vi "UserEventDemo.vi"() -> ()   [LabVIEW 2014]
panel:
  out "progress":i32(slide) scale=0.0..100.0
  out "Msg":string
  in  "ButtonB":bool
  in  "ButtonA":bool
  out "NowTime":timestamp
  out "MsgString":string
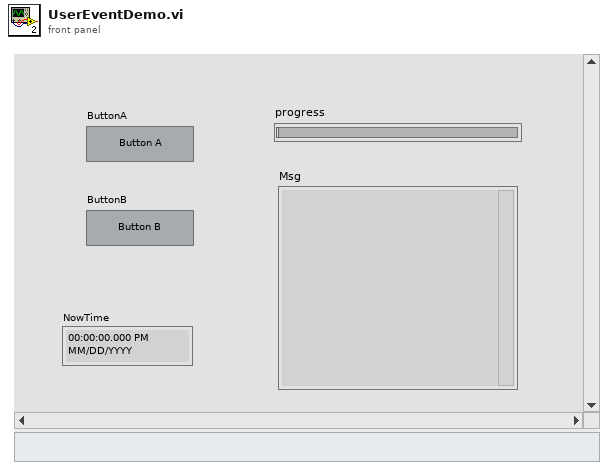
[diagram p1: front panel]
types:
  T1 = cluster{"NowTime":timestamp, "MsgString":string, "UEV":refnum<user-event>}
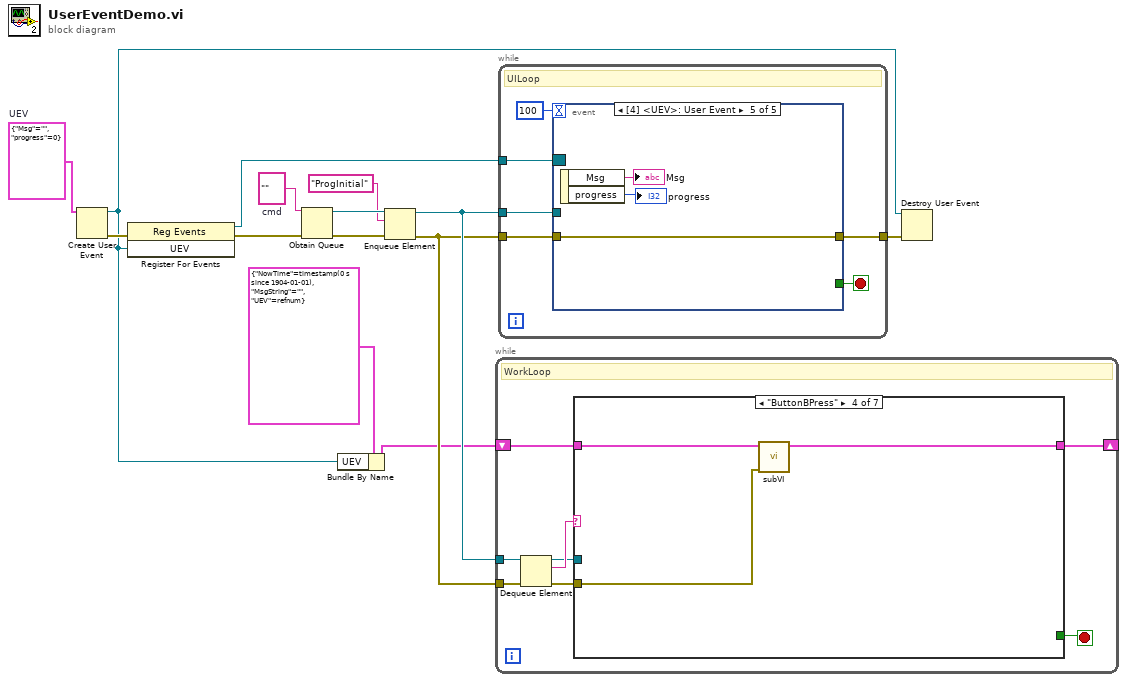
[diagram p0: block diagram]
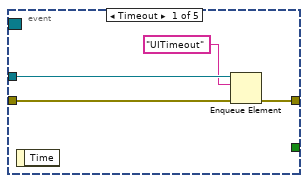
[diagram p2: hidden frame]
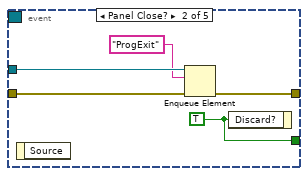
[diagram p3: hidden frame]
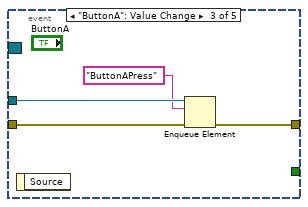
[diagram p4: hidden frame]
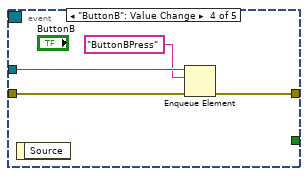
[diagram p5: hidden frame]
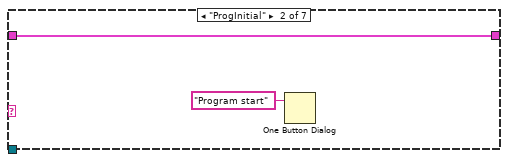
[diagram p7: hidden frame]
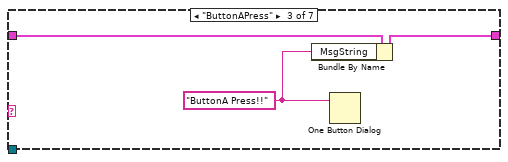
[diagram p8: hidden frame]
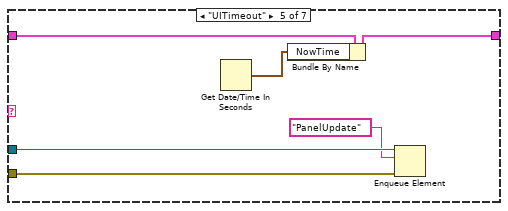
[diagram p9: hidden frame]
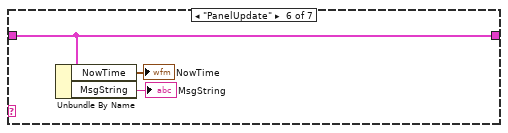
[diagram p10: hidden frame]
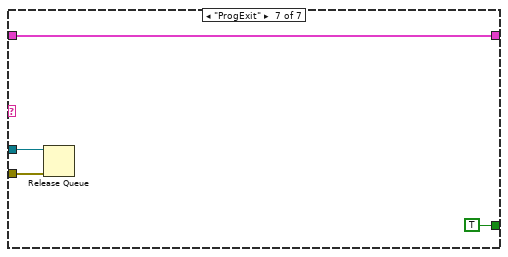
[diagram p11: hidden frame]
diagram:
  w4 = cluster{"Msg":string, "progress":i32} {"Msg"="", "progress"=0}  # UEV
  w12 = ""  # cmd
  n1 = Create User Event(user event datatype=w4) -> (user event=w1:refnum<user-event>, error out=w7:errorcluster)  [unwired: 1 in]
  n2 = register-events(error in=w7, w1) -> (reference out=w5:refnum<event-registration>, error out=w6:errorcluster)  [unwired: 1 in]
  n3 = Obtain Queue(element data type=w12, error in (no error)=w6) -> (queue out=w14:refnum<queue>, error out=w13:errorcluster)  [unwired: 3 in, 1 out]
  n4 = Bundle By Name(cluster=T1 {"NowTime"=timestamp(0 s since 1904-01-01), "MsgString"="", "UEV"=refnum}, "UEV"=w1) -> (w3:T1)
  n5 = Enqueue Element(queue=w14, element="ProgInitial", error in (no error)=w13) -> (queue out=w10:refnum<queue>, error out=w9:errorcluster)  [unwired: 1 in, 1 out]
  n6 = while {
    tunnel: w10 -> [w22]
    tunnel: w9 -> [w21]
    shift-right: [w19] -> _
    shift-left: w3 -> [w18]
    stop <- w15 stop-if-true
    # "WorkLoop"
    n7 = Dequeue Element(queue=w22, error in (no error)=w21) -> (queue out=w17:refnum<queue>, element=w20:string, error out=w16:errorcluster)  [unwired: 1 in, 1 out]
    n8 = case shown="\"ButtonBPress\"" w20 {
      tunnel: [w23 w24 w27 w30 w36 w40 w44] -> w19
      tunnel: w18 -> [w23 w24 w28 w31 w37 w40 w44]
      tunnel: w17 -> [_ _ _ _ w34 _ w43]
      tunnel: w16 -> [_ _ _ w29 w33 _ w42]
      tunnel: [_ _ _ _ _ _ TRUE ("Discard?")] -> w15
      frame Default {
      }
      frame "ProgInitial" {
        n9 = One Button Dialog(message="Program start") -> ()  [unwired: 1 in, 1 out]
      }
      frame "ButtonAPress" {
        w26 = "ButtonA Press!!" ("message")
        n10 = Bundle By Name(cluster=w28, "MsgString"=w26) -> (w27:T1)
        n11 = One Button Dialog(message=w26) -> ()  [unwired: 1 in, 1 out]
      }
      frame "ButtonBPress" {
        n12 = call "subVI.vi"("error in (no error)"=w29, "Cluster in"=w31) -> ("Cluster out"=w30:T1)  [unwired: 9 in]
      }
      frame "UITimeout" {
        n13 = Get Date/Time In Seconds() -> (seconds since 1Jan1904=w35:timestamp)
        n14 = Bundle By Name(cluster=w37, "NowTime"=w35) -> (w36:T1)
        n15 = Enqueue Element(queue=w34, element="PanelUpdate", error in (no error)=w33) -> ()  [unwired: 1 in, 3 out]
      }
      frame "PanelUpdate" {
        n16 = Unbundle By Name(w40) -> ("NowTime"=→"NowTime":timestamp, "MsgString"=→"MsgString":string)
      }
      frame "ProgExit" {
        n17 = Release Queue(queue=w43, error in (no error)=w42) -> ()  [unwired: 1 in, 3 out]
      }
    }
  }
  n18 = while {
    tunnel: w10 -> [w49]
    tunnel: w9 -> [w48]
    tunnel: w5 -> [w46]
    tunnel: [w45] -> w2
    stop <- w47 stop-if-true
    # "UILoop"
    n19 = event shown="[4] <UEV>: User Event" {
      selector: w46 -> [_ _ _ _ _]
      dyn-events: _ -> [_ _ _ _ _]
      timeout: 100 -> [_ _ _ _ _]
      tunnel: w49 -> [w54 w59 w63 w67 _]
      tunnel: w48 -> [w53 w58 w62 w66 w68]
      tunnel: [_ w57 _ _ _] -> w47
      tunnel: [w51 w55 w60 w64 w68] -> w45
      event Timeout {
        n20 = event-data() -> ()  [unwired: 1 in, 1 out]
        n21 = Enqueue Element(queue=w54, element="UITimeout", error in (no error)=w53) -> (error out=w51:errorcluster)  [unwired: 1 in, 2 out]
      }
      event Panel Close? {
        w57 = TRUE ("Discard?")
        n22 = event-data() -> ()  [unwired: 1 in, 1 out]
        n23 = Enqueue Element(queue=w59, element="ProgExit", error in (no error)=w58) -> (error out=w55:errorcluster)  [unwired: 1 in, 2 out]
        n24 = event-data("Discard?"=w57) -> ()  [unwired: 1 in, 1 out]
      }
      event "ButtonA": Value Change {
        n25 = event-data() -> ()  [unwired: 1 in, 1 out]
        n26 = Enqueue Element(queue=w63, element="ButtonAPress", error in (no error)=w62) -> (error out=w60:errorcluster)  [unwired: 1 in, 2 out]
      }
      event "ButtonB": Value Change {
        n27 = event-data() -> ()  [unwired: 1 in, 1 out]
        n28 = Enqueue Element(queue=w67, element="ButtonBPress", error in (no error)=w66) -> (error out=w64:errorcluster)  [unwired: 1 in, 2 out]
      }
      event User Event {
        n29 = event-data() -> ("Msg"=→"Msg":string, "progress"=→"progress":i32)  [unwired: 1 in]
      }
    }
  }
  n30 = Destroy User Event(user event=w1, error in=w2) -> ()  [unwired: 1 out]
